vi "read multiple params.vi"(8 "error in (no error)":errorcluster, 10 "Parameters":u32[](array[numeric]) format="%.0x", 11 "CL57RS in":refnum<class "CL57RS.lvclass">) -> (0 "error out":errorcluster, 2 "Hex Result":u32[](array[numeric]) format="%.0x", 3 "CL57RS out":refnum<class "CL57RS.lvclass">)   [LabVIEW 2025, in "Motor.lvlib" / "CL57RS.lvclass"]
uses:
  CL57RS.lvclass
  CL57RS.lvclass/CL57RS.ctl
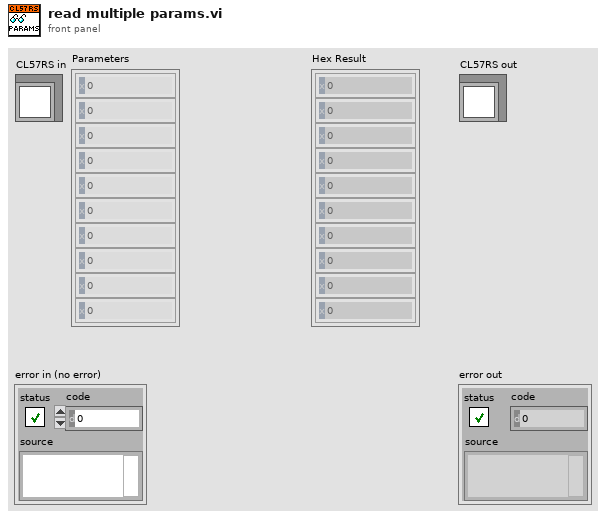
[diagram p1: front panel]
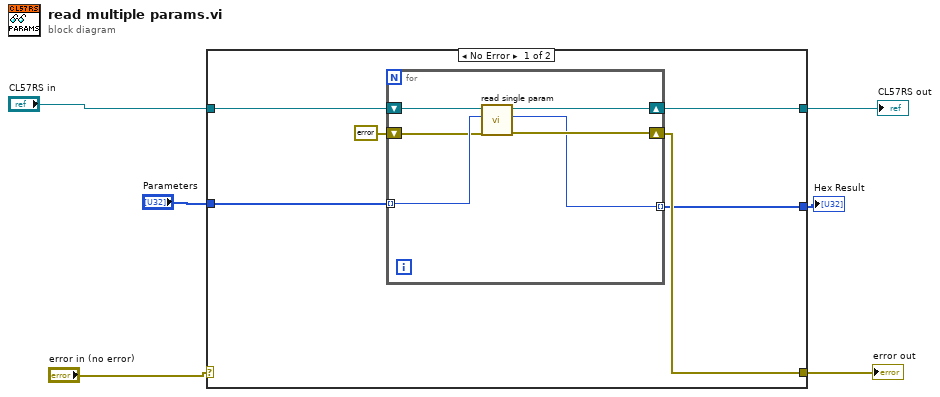
[diagram p0: block diagram]
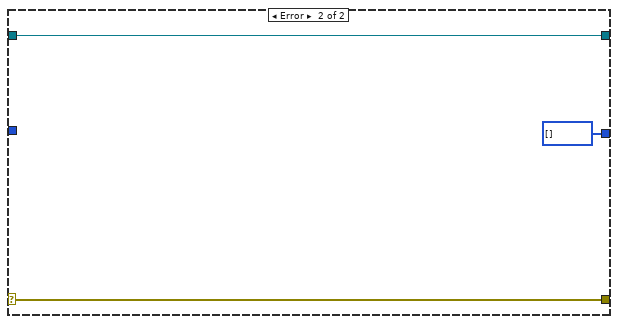
[diagram p2: hidden frame]
diagram:
  n1 = case shown="No Error" "error in (no error)" {
    selector: "error in (no error)" -> [_ w21]
    tunnel: [w10 w21] -> w2
    tunnel: [w9 w20] -> w3
    tunnel: "CL57RS in" -> [w11 w20]
    tunnel: "Parameters" -> [w12 _]
    tunnel: [w8 u16[] []] -> w5
    frame No Error {
      n2 = for {
        tunnel: w12 -> [w17] mode=indexing
        shift-right: [w15] -> w10
        shift-left: errorcluster {"status"=FALSE, "code"=0, "source"=""} ("error out") -> [w16]
        shift-right: [w14] -> w9
        shift-left: w11 -> [w18]
        tunnel: [w13] -> w8 mode=indexing
        n3 = call "read single param.vi"("error in (no error)"=w16, "address"=w17, "CL57RS in"=w18) -> ("error out"=w15:errorcluster, "register"=w13:u16, "CL57RS out"=w14:refnum<class "CL57RS.lvclass">)  [unwired: 6 in]
      }
    }
    frame Error {
    }
  }
  "error out" <- w2
  "CL57RS out" <- w3
  "Hex Result" <- w5
